vi "Configure List Parameters.vi"(0 "VISA resource name":refnum<visa-resource-name>, 1 "Enable Infinite Mode (F: False)":bool, 5 "Repeat Count (0)":u32 max=99 step=1, 7 "List Timing Mode (0:Time)":i32(ring) items=["Time", "Cycle"], 9 "List Sync (0: Immediate)":i32(ring) items=["Immediate", "Phase"], 11 "error in (no error)":errorcluster, 12 "List Phase (0.0 degrees)":dbl min=0.0 max=359.7 format="%.1g") -> (4 "VISA resource name out":refnum<visa-resource-name>, 15 "error out":errorcluster)   [LabVIEW 2018, in "BK Precision 983X Series.lvlib"]
doc: "Configures the list parameters: Infinite mode, repeat count, timing mode, sync mode, and sync phase.\n\nNote: First, run <b>Configure Output Mode.vi</b> to set the instrument to List Moe. Then, run this vi after running <b>Save Recall List Program.vi</b> to recall a list first."
uses:
  <instrlib>/BK Precision 983X Series/BK Precision 983X Series.lvlib
panel:
  # "degree"
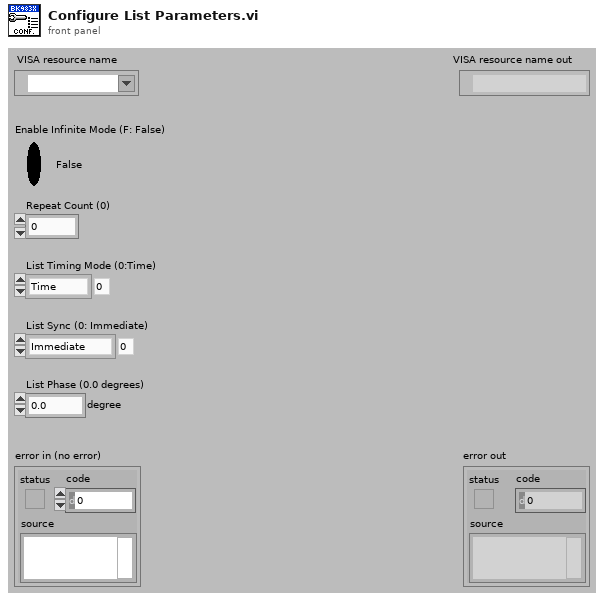
[diagram p1: front panel]
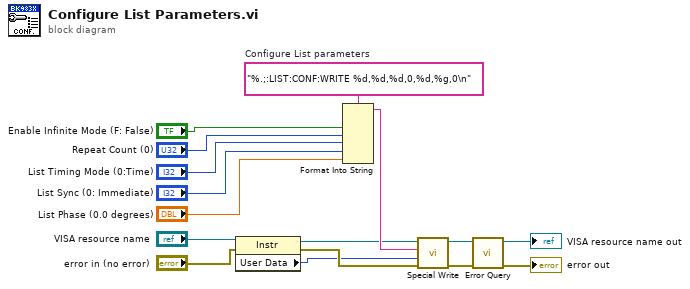
[diagram p0: block diagram]
diagram:
  w14 = "%.;:LIST:CONF:WRITE %d,%d,%d,0,%d,%g,0\n"  # Configure List parameters
  n1 = property class="Instr"(reference="VISA resource name", error in="error in (no error)") -> (reference out=w3:refnum<visa-resource-name>, error out=w2:errorcluster, "User Data"=w1:u32)
  n2 = Format Into String(format string=w14, "Enable Infinite Mode (F: False)", "Repeat Count (0)", "List Timing Mode (0:Time)", "List Sync (0: Immediate)", "List Phase (0.0 degrees)") -> (resulting string=w4:string)  [unwired: 2 in, 1 out]
  n3 = call <instrlib>:"Special Write.vi"("error in (no error)"=w2, "Delay (0 ms)"=w1, "Input String"=w4, "VISA resource name"=w3) -> ("error out"=w5:errorcluster, "VISA resource name out"=w6:refnum<visa-resource-name>)  [unwired: 6 in]
  n4 = call <instrlib>:"Error Query.vi"("error in (no error)"=w5, "VISA resource name"=w6) -> ("error out"=→"error out":errorcluster, "VISA resource name out"=→"VISA resource name out":refnum<visa-resource-name>)  [unwired: 6 in, 2 out]
